vi "CheesyDrive.vi"(6 "Quickturn":bool, 7 "SlowMode":u32, 10 "Wheel":dbl(slide)=-0.023622047244094488 scale=-1.0..1.0, 11 "Throttle":dbl(slide)=0.007874015748031496 scale=-1.0..1.0) -> (2 "Right PWM":dbl, 3 "Left PWM":dbl)   [LabVIEW 2017]
doc: "Implements CheesyDrive. CheesyDrive means that the turn joystick controls the radius of turning instead of the rate of turning. Also implements QuickStop and QuickTurn."
panel:
  in  "ArrayOfSlownesss":T1(array[cluster])=[{"MaxSpeedSlow"=1.0, "SlowRate"=5.0, "MaxTurnSlow"=1.0, "MaxTurnRateSlow"=10.0}, {"MaxSpeedSlow"=0.6, "SlowRate"=4.0, "MaxTurnSlow"=0.8, "MaxTurnRateSlow"=10.0}, {"MaxSpeedSlow"=0.4, "SlowRate"=3.0, "MaxTurnSlow"=0.75, "MaxTurnRateSlow"=10.0}]
  in  "PointsTurn":cluster{"X":dbl, "Y":dbl}[](array[cluster])=[{"X"=0.0, "Y"=0.0}, {"X"=0.04, "Y"=0.0}, {"X"=0.041, "Y"=0.01}, {"X"=1.0, "Y"=1.0}]
  in  "PointsQuickTurn":cluster{"X":dbl, "Y":dbl}[](array[cluster])=[{"X"=0.0, "Y"=0.0}, {"X"=0.04, "Y"=0.0}, {"X"=0.8, "Y"=0.7}, {"X"=1.0, "Y"=1.0}]
  in  "PointsThrottle":cluster{"X":dbl, "Y":dbl}[](array[cluster])=[{"X"=0.0, "Y"=0.0}, {"X"=0.04, "Y"=0.0}, {"X"=0.0251, "Y"=0.15}, {"X"=1.0, "Y"=1.0}]
  in  "QSMult":dbl=0.15
  in  "WheelNonLinearity":dbl=0.65
  in  "negInertiaScalar":dbl=3.0
  in  "alpha":dbl=0.1
  out "QuickStop Value":dbl(graph)
  in  "Sensitivty":dbl=1.0
  # "These are the inputs and outputs\nNot configuration"
  # "Check block diagram for details on these"
  # "normal"
  # "Switch"
  # "Scale"
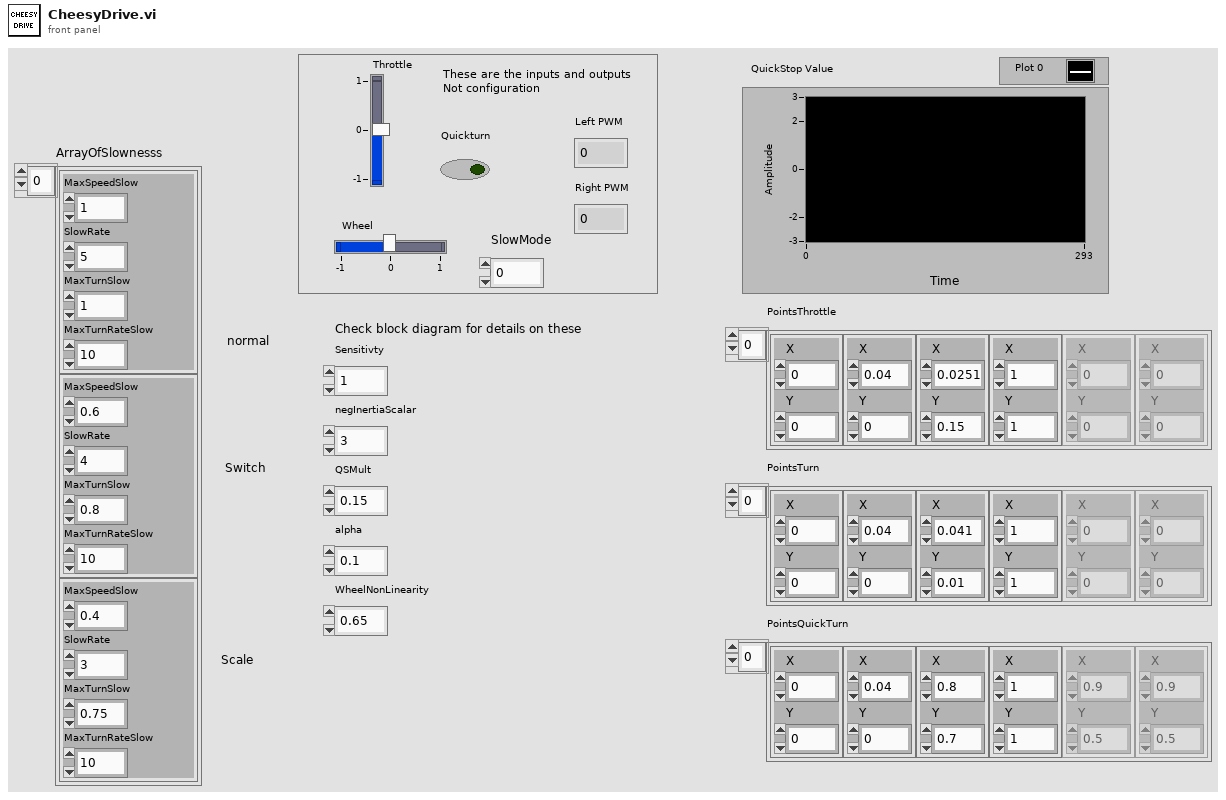
[diagram p1: front panel]
types:
  T1 = cluster{"MaxSpeedSlow":dbl, "SlowRate":dbl, "MaxTurnSlow":dbl, "MaxTurnRateSlow":dbl}[]
  T2 = cluster{"MaxSpeedSlow":dbl, "SlowRate":dbl, "MaxTurnSlow":dbl, "MaxTurnRateSlow":dbl}
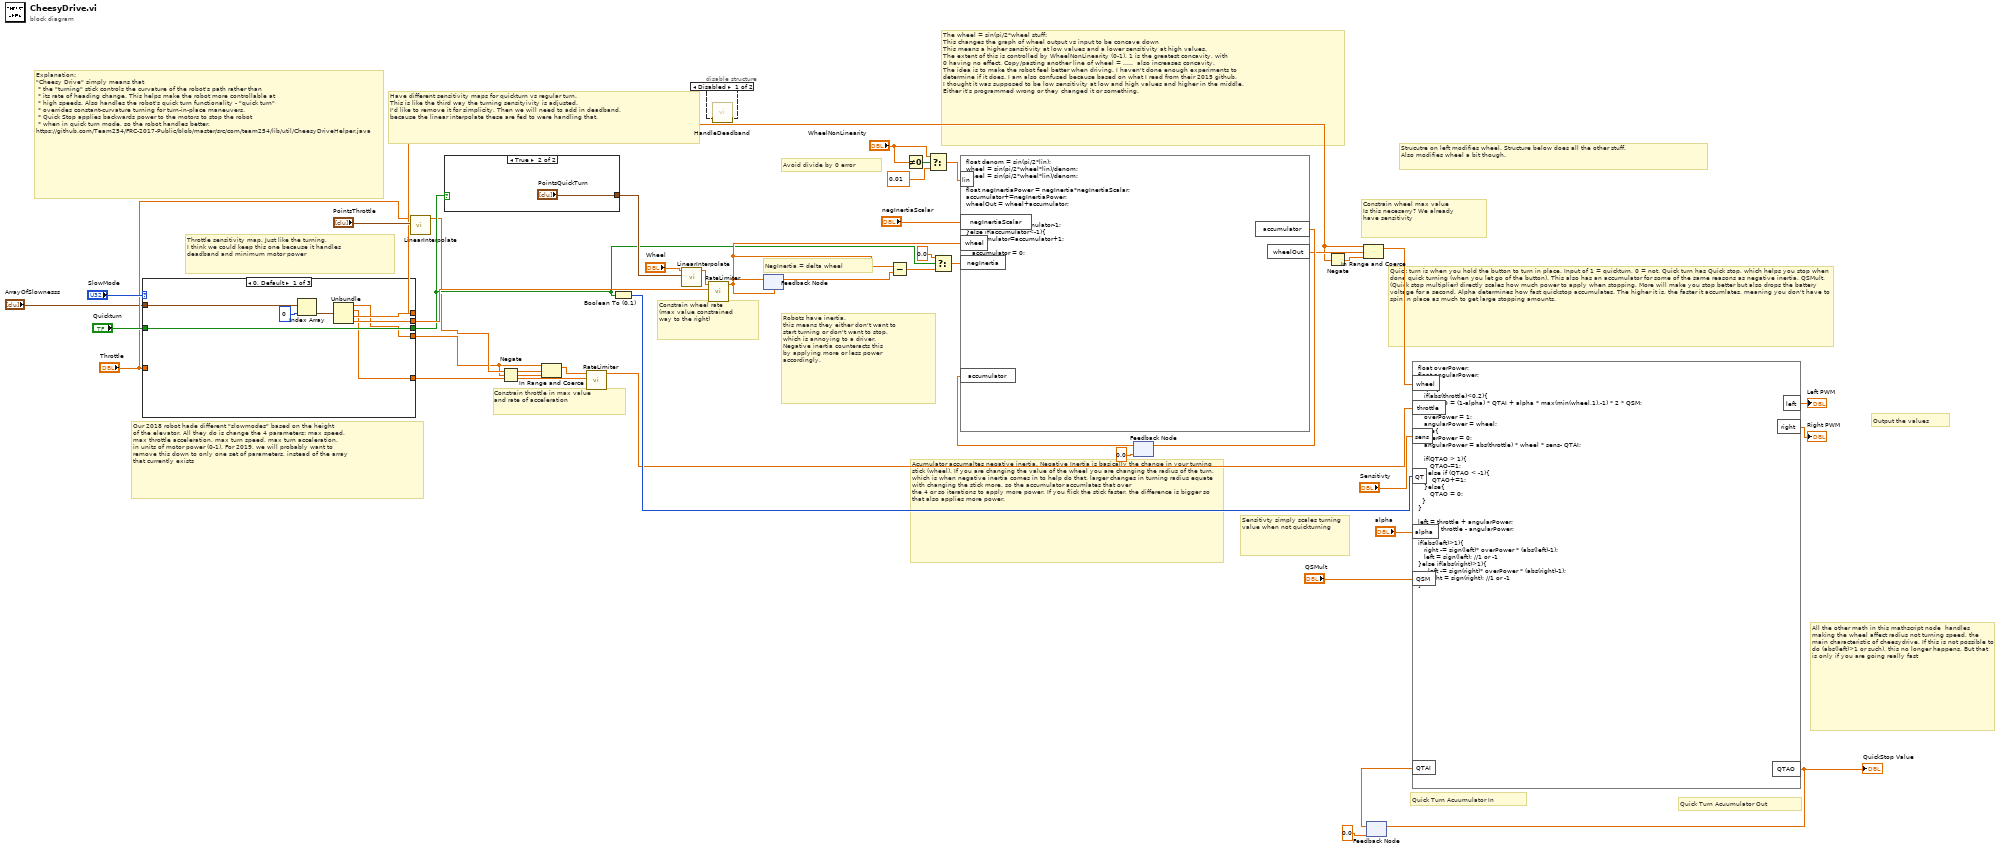
[diagram p0: block diagram]
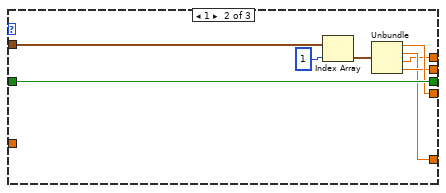
[diagram p3: hidden frame]
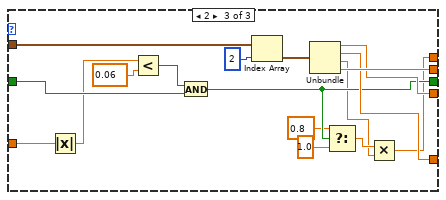
[diagram p4: hidden frame]
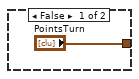
[diagram p5: hidden frame]
diagram:
  # "Strucutre on left modifies wheel. Structure below does all the other stuff.\nAlso modifies wheel a bit though."
  # "Sensitivty simply scales turning value when not quickturning"
  # "All the other math in this mathscript node  handles making the wheel affect radius not turning speed, the main characteristic of cheesydrive. If this is not possible to do (abs(left)>1 or such), this no longer happens. But that is only if you are going really fast"
  # "Quick turn is when you hold the button to turn in place. Input of 1 = quickturn, 0 = not. Quick turn has Quick stop, which helps you stop when done quick turning (when you let go of the button). This also has an accumulator for some of the same reasons as negative inertia. QSMult, (Quick stop multiplier) directly scales how much power to apply when stopping. More will make you stop better but also drops the battery voltage for a second. Alpha determines how fast quickstop accumulates. The higher it is, the faster it accumlates, meaning you don't have to spin in place as much to get large stopping amounts."
  # "Output the values"
  # "Acumulator accumaltes negative inertia. Negative Inertia is basically the change in your turning stick (wheel). If you are changing the value of the wheel you are changing the radius of the turn, which is when negative inertia comes in to help do that. larger changes in turning radius equate with changing the stick more, so the accumulator accumlates that over\nthe 4 or so iterations to apply more power. If you flick the stick faster, the difference is bigger so that also applies more power."
  # "The wheel = sin(pi/2*wheel stuff:\nThis changes the graph of wheel output vs input to be concave down\nThis means a higher sensitivity at low values and a lower sensitivity at high values.\nThe extent of this is controlled by WheelNonLinearity (0-1). 1 is the greatest concavity, with\n0 having no effect. Copy/pasting another line of wheel = .....  also increases concavity.\nThe idea is to make the robot feel better when driving. I haven't done enough experiments to \ndetermine if it does. I am also confused because based on what I read from their 2015 github,\nI thought it was supposed to be low sensitivity at low and high values and higher in the middle.\nEither it's programmed wrong or they changed it or something."
  # "Constrain wheel max value\nIs this necesarry? We already\nhave sensitivity"
  # "Constrain wheel rate\n(max value constrained\nway to the right)"
  # "Throttle sensitivity map. Just like the turning,\nI think we could keep this one because it handles\ndeadband and minimum motor power"
  # "Have different sensitivity maps for quickturn vs regular turn.\nThis is like the third way the turning sensityivity is adjusted. \nI'd like to remove it for simplicity. Then we will need to add in deadband,\nbecause the linear interpolate these are fed to were handling that."
  # "Robots have inertia.\nthis means they either don't want to\nstart turning or don't want to stop,\nwhich is annoying to a driver. \nNegative inertia counteracts this\nby applying more or less power\naccordingly."
  # "Constrain throttle in max value\nand rate of acceleration"
  # "Our 2018 robot hade different \"slowmodes\" based on the height\nof the elevator. All they do is change the 4 parameters: max speed,\nmax throttle acceleration, max turn speed, max turn acceleration,\nin units of motor power (0-1). For 2019, we will probably want to\nremove this down to only one set of parameters, instead of the array\nthat currently exists"
  # "Avoid divide by 0 error"
  # "NegInertia = delta wheel"
  # "Explanation:\n\"Cheesy Drive\" simply means that\n * the \"turning\" stick controls the curvature of the robot's path rather than\n * its rate of heading change. This helps make the robot more controllable at\n * high speeds. Also handles the robot's quick turn functionality - \"quick turn\"\n * overrides constant-curvature turning for turn-in-place maneuvers.\n * Quick Stop applies backwards power to the motors to stop the robot\n * when in quick turn mode, so the robot handles better.\nhttps://github.com/Team254/FRC-2017-Public/blob/master/src/com/team254/lib/util/CheesyDriveHelper.java"
  # "Quick Turn Acuumulator Out"
  # "Quick Turn Acuumulator In"
  n1 = case shown="0, Default" "SlowMode" {
    tunnel: [w43 w52 w66] -> w21
    tunnel: [w44 w54 w68] -> w5
    tunnel: [w45 w51 w59] -> w19
    tunnel: [w46 w53 w69] -> w17
    tunnel: "Quickturn" -> [w50 w58 w75]
    tunnel: [w50 w58 w63] -> w10
    tunnel: "Throttle" -> [_ _ w67]
    tunnel: "ArrayOfSlownesss" -> [w47 w55 w72]
    frame 0, Default {
      n2 = Index Array(array=w47, index=0) -> (element=w48:T2)
      n3 = Unbundle(w48) -> ("MaxSpeedSlow"=w44:dbl, "SlowRate"=w43:dbl, "MaxTurnSlow"=w45:dbl, "MaxTurnRateSlow"=w46:dbl)
    }
    frame 1 {
      n4 = Index Array(array=w55, index=1) -> (element=w56:T2)
      n5 = Unbundle(w56) -> ("MaxSpeedSlow"=w54:dbl, "SlowRate"=w52:dbl, "MaxTurnSlow"=w51:dbl, "MaxTurnRateSlow"=w53:dbl)
    }
    frame 2 {
      n6 = Absolute Value(x=w67) -> (abs(x)=w65:dbl)
      n7 = Less?(x=w65, y=0.06) -> (x < y?=w74:bool)
      n8 = And(x=w74, y=w75) -> (x .and. y?=w63:bool)
      n9 = Index Array(array=w72, index=2) -> (element=w70:T2)
      n10 = Unbundle(w70) -> ("MaxSpeedSlow"=w68:dbl, "SlowRate"=w66:dbl, "MaxTurnSlow"=w60:dbl, "MaxTurnRateSlow"=w69:dbl)
      n11 = Select(t=0.8, s=w63, f=1.0) -> (s? t:f=w61:dbl)
      n12 = Multiply(x=w61, y=w60) -> (x*y=w59:dbl)
    }
  }
  n13 = call "LinearInterpolate.vi"("Points"="PointsThrottle", "Value"="Throttle") -> ("Output"=w7:dbl)  [unwired: 9 in]
  n14 = case shown="True" w10 {
    tunnel: ["PointsTurn" "PointsQuickTurn"] -> w23
    frame False {
    }
    frame True {
    }
  }
  n15 = Negate(x=w5) -> (-x=w6:dbl)
  n16 = In Range and Coerce(upper limit=w5, x=w7, lower limit=w6) -> (coerced(x)=w8:dbl)  [unwired: 1 out]
  n17 = call "RateLimiter.vi"("Max dx/dt"=w21, "Input"=w8) -> ("Output"=w36:dbl)  [unwired: 9 in]
  n18 = Boolean To (0,1)(Boolean=w10) -> (0, 1=w40:i16)
  n19 = call "LinearInterpolate.vi"("Points"=w23, "Value"="Wheel") -> ("Output"=w18:dbl)  [unwired: 9 in]
  n20 = disable-structure shown="Disabled" {
    frame Disabled {
      n21 = call "HandleDeadband.vi"() -> ()  [unwired: 11 in, 1 out]
    }
    frame Enabled {
    }
  }
  n22 = call "RateLimiter.vi"("Max dx/dt"=w17, "Input"=w18) -> ("Output"=w25:dbl)  [unwired: 9 in]
  n23 = feedback #1(w25) -> (w33:dbl)
  n24 = feedback-in #1(w25) -> ()
  n25 = Subtract(x=w25, y=w33) -> (x-y=w15:dbl)
  n26 = Not Equal To 0?(x="WheelNonLinearity") -> (x != 0?=w4:bool)
  n27 = Select(t="WheelNonLinearity", s=w4, f=0.01) -> (s? t:f=w1:dbl)
  n28 = Select(t=0.0, s=w10, f=w15) -> (s? t:f=w16:dbl)
  n29 = feedback #2(0.0 ("Wheel")) -> (w32:dbl)
  n30 = formula code="float denom = sin(pi/2*lin);\nwheel = sin(pi/2*wheel*lin)/denom;\nwheel = sin(pi/2*wheel*lin)/denom;\n\nfloat negInertiaPower = negInertia*negInertiaScalar;\naccumulator+=negInertiaPower;\nwheelOut = wheel+accumulator;\n\nif(accumulator>1){\n   accumulator=accumulator-1;\n}else if(accumulator<-1){\n   accumulator=accumulator+1;\n}else{\n   accumulator = 0;\n}"("wheel"=w25, "negInertia"=w16, "accumulator"=w32, "negInertiaScalar"="negInertiaScalar", "lin"=w1) -> ("accumulator"=w30:dbl, "wheelOut"=w27:dbl)
  n31 = feedback-in #2(w30) -> ()
  n32 = Negate(x=w19) -> (-x=w20:dbl)
  n33 = In Range and Coerce(upper limit=w19, x=w27, lower limit=w20) -> (coerced(x)=w28:dbl)  [unwired: 1 out]
  n34 = feedback #3(0.0 ("QTAccumulatorO")) -> (w38:dbl)
  n35 = formula code="float overPower;\nfloat angularPower;\n\nif(QT){\n   if(abs(throttle)<0.2){\n      QTAO = (1-alpha) * QTAI + alpha * max(min(wheel,1),-1) * 2 * QSM;\n   }\n   overPower = 1;\n   angularPower = wheel;\n}else{\n   overPower = 0;\n   angularPower = abs(throttle) * wheel * sens- QTAI;\n\n   if(QTAO > 1){\n      QTAO-=1;\n   }else if (QTAO < -1){\n       QTAO+=1;\n   }else{\n      QTAO = 0;\n  }\n}\n\nleft = throttle + angularPower;\nright = throttle - angularPower;\n\nif(abs(left)>1){\n   right -= sign(left)* overPower * (abs(left)-1);\n   left = sign(left); //1 or -1\n}else if(abs(right)>1){\n     left -= sign(right)* overPower * (abs(right)-1);\n     right = sign(right); //1 or -1 \n}"("wheel"=w28, "throttle"=w36, "sens"="Sensitivty", "QT"=w40, "alpha"="alpha", "QTAI"=w38, "QSM"="QSMult") -> ("left"=→"Left PWM":dbl, "right"=→"Right PWM":dbl, "QTAO"=w41:dbl)
  "QuickStop Value" <- w41
  n36 = feedback-in #3(w41) -> ()
